vi "Execute.vi"(8 "error in (no error)":errorcluster, 9 "System in":refnum<class "System.lvclass">, 10 "Command in":refnum<class "Command.lvclass">, 11 "CT-Energizing-State in":refnum<class "CT-Energizing-State.lvclass">) -> (0 "error out":errorcluster, 2 "Next State":refnum<class "State.lvclass">, 3 "CT-Energizing-State out":refnum<class "CT-Energizing-State.lvclass">)   [LabVIEW 2013, in "CT-Energizing-State.lvclass"]
uses:
  CT-Energizing-State.lvclass
  Commands/Command/Command.lvclass
  Systems/System/System.lvclass
  State/State.lvclass
  Systems/Catapult/Catapult.lvclass
  CT-Energized-State/CT-Energized-State.lvclass
  Robot Global Data.vi
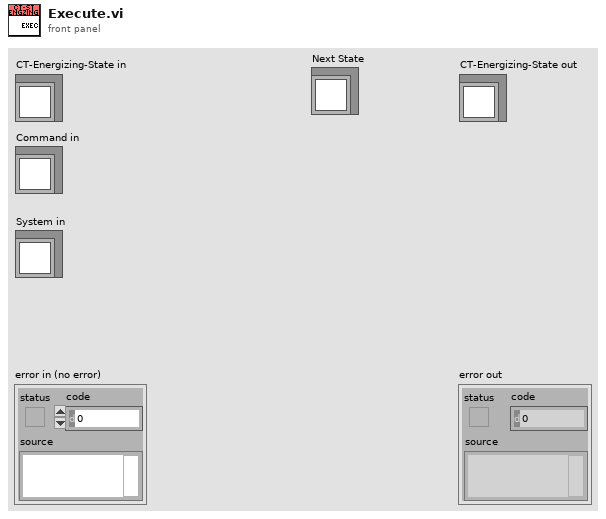
[diagram p1: front panel]
types:
  T1 = typedef "WPI_DigitalInputDevRef.ctl" = cluster{"DevStatus":errorcluster, "DIO Channel":T2, "Digital Module":T3}
  T2 = typedef "FPGA_DIOChannel.ctl" = enum8{"DIO 1", "DIO 2", "DIO 3", "DIO 4", "DIO 5", "DIO 6", "DIO 7", "DIO 8", "DIO 9", "DIO 10", "DIO 11", "DIO 12", "DIO 13", "DIO 14", "Invalid"}
  T3 = typedef "FPGA_TypedefDigitalModule.ctl" = enum16{"Digital Module 1", "Digital Module 2"}
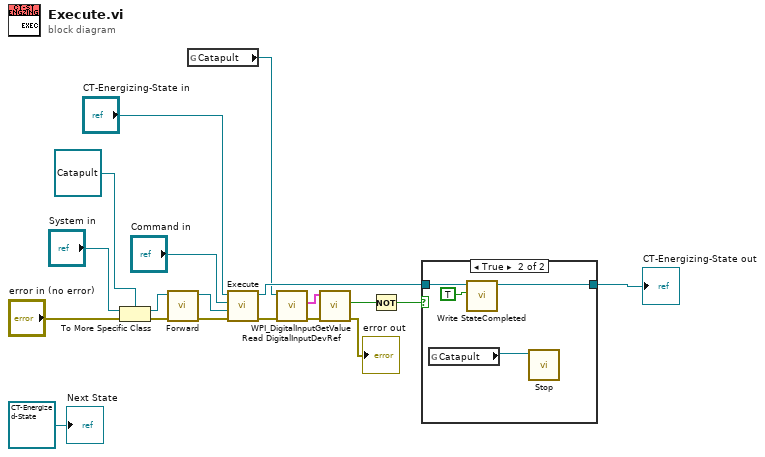
[diagram p0: block diagram]
diagram:
  n1 = To More Specific Class(target class=refnum<class "Catapult.lvclass"> refnum ("Catapult.lvclass"), reference="System in", error in="error in (no error)") -> (specific class reference=w13:refnum<class "Catapult.lvclass">, error out=w14:errorcluster)
  n2 = call-dynamic "Forward.vi"("error in (no error)"=w14, "Catapult in"=w13) -> ("error out"=w6:errorcluster, "Catapult out"=w7:refnum<class "Catapult.lvclass">)  [unwired: 8 in]
  n3 = global read "Robot Global Data.vi" "Catapult"() -> (w5:refnum<class "Catapult.lvclass">)
  n4 = call-parent "Execute.vi"("error in (no error)"=w6, "System in"=w7, "Command in"="Command in", "State in"="CT-Energizing-State in") -> ("error out"=w2:errorcluster, "State out"=w10:refnum<class "CT-Energizing-State.lvclass">)  [unwired: 5 in, 1 out]
  n5 = call-dynamic "Read DigitalInputDevRef.vi"("error in (no error)"=w2, "Catapult in"=w5) -> ("error out"=w11:errorcluster, "DigitalInputDevRef"=w12:T1)  [unwired: 7 in, 1 out]
  n6 = call <vilib>:"WPI_DigitalInputGetValue.vi"("error in (no error)"=w11, "DigitalInputDevRef"=w12) -> ("error out"=→"error out":errorcluster, "Value"=w4:bool)  [unwired: 7 in, 1 out]
  n7 = Not(x=w4) -> (.not. x?=w3:bool)
  n8 = case shown="True" w3 {
    tunnel: w10 -> [w20 w23]
    tunnel: [w20 w22] -> w9
    frame False {
    }
    frame True {
      n9 = global read "Robot Global Data.vi" "Catapult"() -> (w21:refnum<class "Catapult.lvclass">)
      n10 = call-dynamic "Write StateCompleted.vi"("StateCompleted"=TRUE, "State in"=w23) -> ("State out"=w22:refnum<class "CT-Energizing-State.lvclass">)  [unwired: 8 in, 1 out]
      n11 = call-dynamic "Stop.vi"("Catapult in"=w21) -> ()  [unwired: 9 in, 2 out]
    }
  }
  "CT-Energizing-State out" <- w9
  "Next State" <- refnum<class "CT-Energized-State.lvclass"> refnum ("CT-Energized-State.lvclass")
